vi "Data Type to Test Executive.vi"(8 "error in (no error)":errorcluster, 11 "Data Type":refnum<class "Data Type.lvclass">) -> (0 "error out":errorcluster, 3 "Test Executive Ref":refnum<data-value>)   [LabVIEW 2017, in "Custom Type Test Executive.lvlib" / "Test Executive.lvclass"]
uses:
  <vilib>/gpm_packages/@cs/test-executive/Source/Custom Type Test Executive/Test Executive Data Type/Test Executive.lvclass
  <vilib>/gpm_packages/@cs/test-executive/Source/Test Executive/ITestExecutive/ITest Executive.lvclass
  <vilib>/gpm_packages/@cs/data-type-serializer/source/Data Type/Data Type.lvclass
  <vilib>/gpm_packages/@cs/test-executive/Source/Custom Type Test Executive/Test Executive Data Type/Test Executive.lvclass/Test Executive.ctl
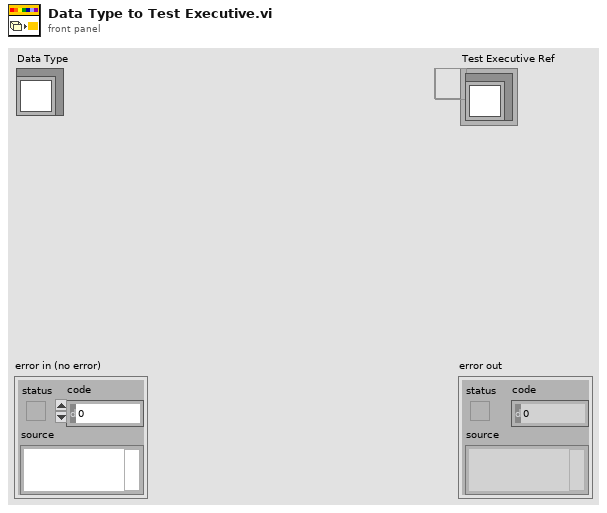
[diagram p1: front panel]
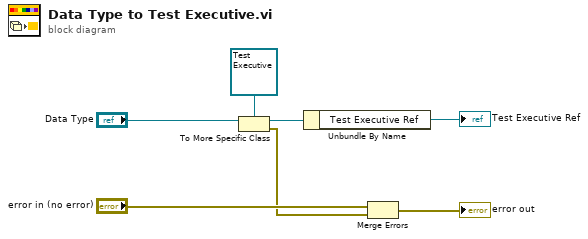
[diagram p0: block diagram]
diagram:
  n1 = To More Specific Class(target class=refnum<class "Test Executive.lvclass"> refnum ("Boolean out"), reference="Data Type") -> (specific class reference=w4:refnum<class "Test Executive.lvclass">, error out=w1:errorcluster)  [unwired: 1 in]
  n2 = Unbundle By Name(w4) -> ("Test Executive Ref"=→"Test Executive Ref":refnum<data-value>)
  n3 = Merge Errors("error in (no error)", w1) -> (→"error out":errorcluster)
